vi "get Broadcast Ping Result.vi"(8 "error in (no error)":errorcluster, 9 "id":i32, 10 "protocol_version":i32, 11 "port_num":i32) -> (0 "error out":errorcluster, 3 "function return":u8)   [LabVIEW 2018, in "labview.lvlib"]
doc: "WINDECLSPEC uint8_t getBroadcastPingResult (int port_num, int protocol_version, int id);"
uses:
  labview.lvlib
  dxl_x86_c.dll
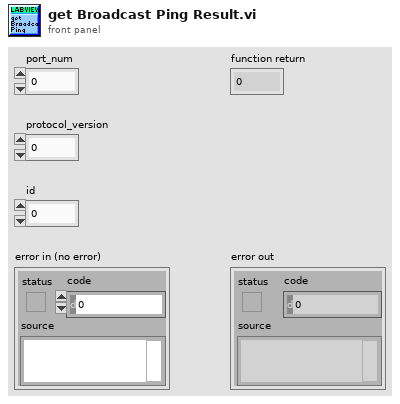
[diagram p1: front panel]
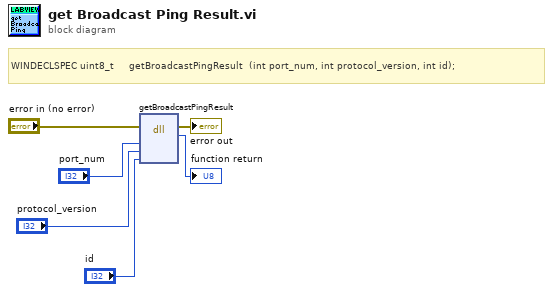
[diagram p0: block diagram]
diagram:
  # "WINDECLSPEC uint8_t     getBroadcastPingResult  (int port_num, int protocol_version, int id);"
  n1 = dll-call lib="C:/Users/joaos/OneDrive/Documents/[PhD]/Project Omnidirectional Vehicle/Vanes/LabView_code/joaoandthethreestands/DynamixelSDK-3.7.31/labview/new_compilation/dxl_x86_c.*" fn="getBroadcastPingResult"(error in="error in (no error)", "port_num"="port_num", "protocol_version"="protocol_version", "id"="id") -> (error out=→"error out":errorcluster, →"function return":u8)  [unwired: 5 in, 1 out]
